vi "TokenizeString.vi"(2 "Delimiter array":string[](array[string])=[","], 3 "String to be tokenized":string="5101,5102,5103,5104,5105,5106") -> (0 "Output array":string[](array[string]))   [LabVIEW 2012]
doc: "Takes in input string and an array of delimiter strings.\nTokenizes the string.\nOutputs an array of strings, comprised of those characters between the delimiters."
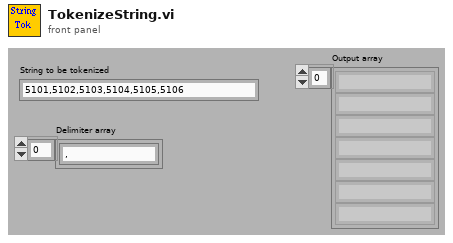
[diagram p1: front panel]
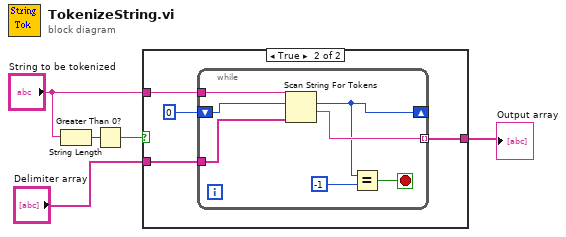
[diagram p0: block diagram]
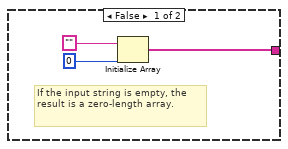
[diagram p2: hidden frame]
diagram:
  n1 = String Length(string="String to be tokenized") -> (length=w2:i32)
  n2 = Greater Than 0?(x=w2) -> (x > 0?=w1:bool)
  n3 = case shown="True" w1 {
    tunnel: "String to be tokenized" -> [_ w11]
    tunnel: "Delimiter array" -> [_ w10]
    tunnel: [w6 w9] -> w4
    frame False {
      # "If the input string is empty, the result is a zero-length array."
      n4 = Initialize Array("", 0) -> (w6:string[])
    }
    frame True {
      n5 = while {
        shift-right: [w13] -> _
        shift-left: 0 -> [w19]
        tunnel: w11 -> [w17]
        tunnel: w10 -> [w16]
        tunnel: [w15] -> w9 mode=indexing
        stop <- w18 stop-if-true
        n6 = Scan String For Tokens(6:w16, 8:w19, 9:w17) -> (1:w15:string, 2:w13:i32)  [unwired: 3 in, 2 out]
        n7 = Equal?(x=w13, y=-1) -> (x = y?=w18:bool)
      }
    }
  }
  "Output array" <- w4
